vi "Guess Current With Offset.vi"(7 "V or I?":enum16{"Voltage", "Current"}(ring), 8 "error in (no error)":errorcluster, 9 "Offset":dbl, 10 "Desired Field":dbl, 11 "Magna Power in":refnum<class "Magna Power.lvclass">) -> (0 "error out":errorcluster, 2 "Guess":dbl, 3 "Magna Power out":refnum<class "Magna Power.lvclass">)   [LabVIEW 2012, in "Magna Power.lvclass"]
doc: "This VI is for use in scanning the current only. It finds the current necessary to create a desired field from the lookup table, and then it adds to that current value an offset. This is so we don't have to calibrate the magnet each scan.\n\nKyle Miller, Jun 2014"
uses:
  Magna Power.lvclass
  Magna Power.lvclass/Magna Power.ctl
  Magna Power Constants.vi
  <vilib>/gmath/NI_Gmath.lvlib
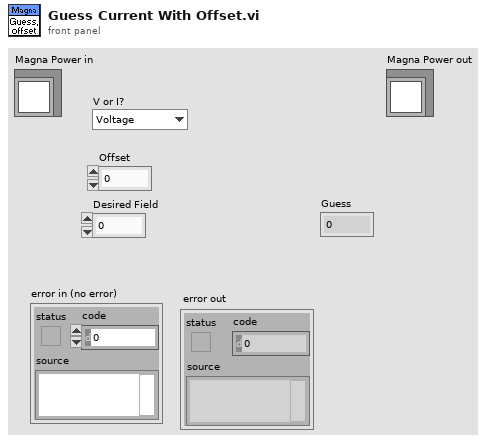
[diagram p1: front panel]
types:
  T1 = cluster{"Magna Voltage":dbl[], "Magna Current":dbl[], "Magnetic Field":dbl[], "Fluke Voltage":dbl[]}
  T2 = cluster{"Magna Current":dbl[], "Magnetic Field":dbl[], "Fluke Voltage":dbl[]}
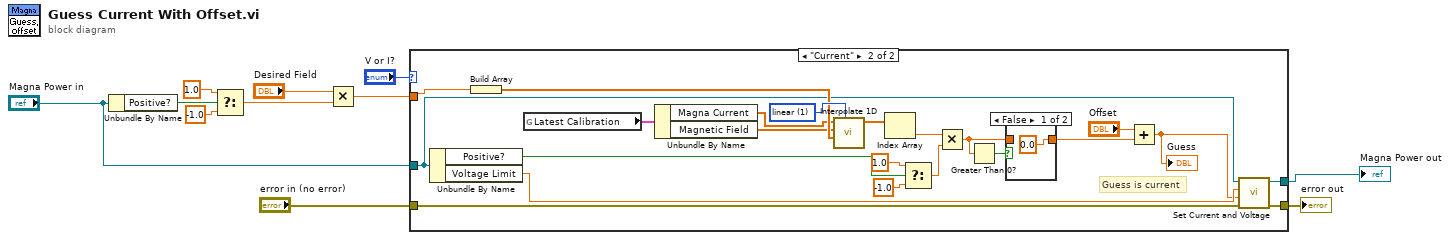
[diagram p0: block diagram]
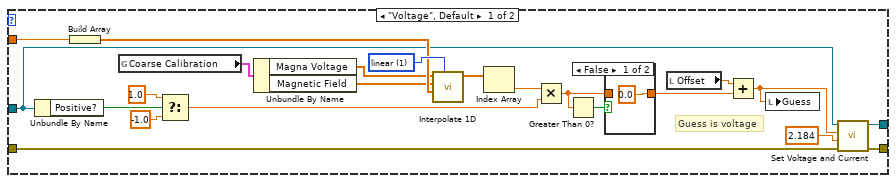
[diagram p2: hidden frame]
diagram:
  n1 = Unbundle By Name("Magna Power in") -> ("Positive?"=w11:bool)
  n2 = Select(t=1.0, s=w11, f=-1.0) -> (s? t:f=w8:dbl)
  n3 = Multiply(x="Desired Field", y=w8) -> (x*y=w7:dbl)
  n4 = case shown="\"Current\"" "V or I?" {
    tunnel: w7 -> [w19 w57]
    tunnel: [w12 w39] -> w5
    tunnel: "Magna Power in" -> [w15 w38]
    tunnel: [w13 w40] -> w2
    tunnel: "error in (no error)" -> [w14 w41]
    frame "Voltage", Default {
      w32 = 1 items=["nearest", "linear", "spline", "cubic Hermite", "Lagrange"] ("method")
      # "Guess is voltage"
      n5 = Unbundle By Name(w15) -> ("Positive?"=w24:bool)
      n6 = Build Array(w19) -> (w31:dbl[])
      n7 = global read "Magna Power Constants.vi" "Coarse Calibration"() -> (w33:T1)
      n8 = Select(t=1.0, s=w24, f=-1.0) -> (s? t:f=w22:dbl)
      n9 = Unbundle By Name(w33) -> ("Magna Voltage"=w28:dbl[], "Magnetic Field"=w29:dbl[])
      n10 = call <vilib>:"Interpolate 1D.vi"("method"=w32, "xi"=w31, "X"=w29, "Y"=w28) -> ("yi"=w30:dbl[])  [unwired: 5 in, 2 out]
      n11 = Index Array(array=w30) -> (element=w23:dbl)  [unwired: 1 in]
      n12 = Multiply(x=w23, y=w22) -> (x*y=w21:dbl)
      n13 = Greater Than 0?(x=w21) -> (x > 0?=w27:bool)
      n14 = case shown="False" w27 {
        tunnel: [0.0 ("Numeric") w35] -> w20
        tunnel: w21 -> [_ w35]
        frame False {
        }
        frame True {
        }
      }
      n15 = local read "Offset"() -> (w18:dbl)
      n16 = Add(x=w18, y=w20) -> (x+y=w16:dbl)
      n17 = local write "Guess"(w16) -> ()
      n18 = call "Set Voltage and Current.vi"("error in (no error)"=w14, "Current Limit"=2.184, "Voltage Limit"=w16, "Magna Power in"=w15) -> ("error out"=w13:errorcluster, "Magna Power out"=w12:refnum<class "Magna Power.lvclass">)  [unwired: 6 in]
    }
    frame "Current" {
      w55 = 1 items=["nearest", "linear", "spline", "cubic Hermite", "Lagrange"] ("method")
      # "Guess is current"
      n19 = Unbundle By Name(w38) -> ("Positive?"=w47:bool, "Voltage Limit"=w37:dbl)
      n20 = Build Array(w57) -> (w54:dbl[])
      n21 = global read "Magna Power Constants.vi" "Latest Calibration"() -> (w56:T2)
      n22 = Unbundle By Name(w56) -> ("Magna Current"=w51:dbl[], "Magnetic Field"=w52:dbl[])
      n23 = call <vilib>:"Interpolate 1D.vi"("method"=w55, "xi"=w54, "X"=w52, "Y"=w51) -> ("yi"=w53:dbl[])  [unwired: 5 in, 2 out]
      n24 = Index Array(array=w53) -> (element=w46:dbl)  [unwired: 1 in]
      n25 = Select(t=1.0, s=w47, f=-1.0) -> (s? t:f=w45:dbl)
      n26 = Multiply(x=w46, y=w45) -> (x*y=w44:dbl)
      n27 = Greater Than 0?(x=w44) -> (x > 0?=w50:bool)
      n28 = case shown="False" w50 {
        tunnel: [0.0 ("Numeric") w59] -> w42
        tunnel: w44 -> [_ w59]
        frame False {
        }
        frame True {
        }
      }
      n29 = Add(x="Offset", y=w42) -> (x+y=w36:dbl)
      "Guess" <- w36
      n30 = call "Set Current and Voltage.vi"("error in (no error)"=w41, "Current Limit"=w36, "Voltage Limit"=w37, "Magna Power in"=w38) -> ("error out"=w40:errorcluster, "Magna Power out"=w39:refnum<class "Magna Power.lvclass">)  [unwired: 6 in]
    }
  }
  "Magna Power out" <- w5
  "error out" <- w2
